vi "Stop Core.vi"(10 "final error code":i32, 11 "VF Device Selection in":refnum<class "VF Device Selection.lvclass">) -> (3 "VF Device Selection out":refnum<class "VF Device Selection.lvclass">)   [LabVIEW 2018, in "VF Device Selection Actor.lvlib" / "VF Device Selection.lvclass"]
doc: "(<B>Filename</B>: Actor Framework.lvlib:Actor.lvclass:Stop Core.vi)\n\nDefines what the actor does before it stops. Use the <B>final error code</B> input to determine whether the actor shut down in response to an error.\n\nBy default, this method does nothing. A descendant class may override it to define behavior, such as shutting down any processes the actor initiated in its override of the Actor Core method."
uses:
  VF Device Selection.lvclass
  VF Device Selection.lvclass/VF Device Selection.ctl
  <vilib>/ActorFramework/Actor/Actor.lvclass
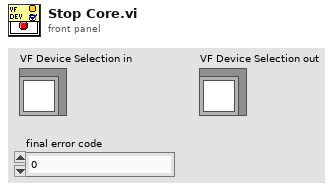
[diagram p1: front panel]
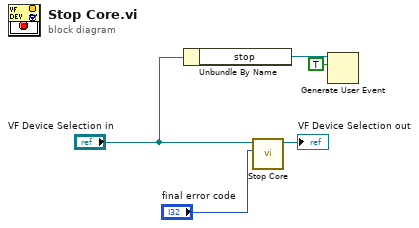
[diagram p0: block diagram]
diagram:
  n1 = Unbundle By Name("VF Device Selection in") -> ("stop"=w2:refnum<user-event>)
  n2 = call-parent "Stop Core.vi"("final error code"="final error code", "Actor in"="VF Device Selection in") -> ("Actor out"=→"VF Device Selection out":refnum<class "VF Device Selection.lvclass">)  [unwired: 9 in]
  n3 = Generate User Event(user event=w2, event data cluster=TRUE ("event data")) -> ()  [unwired: 2 in, 2 out]
